vi "Init.vi"(8 "error in":errorcluster, 11 "object in":refnum<class "Camera Imaqdx CFG.lvclass">) -> (0 "error out":errorcluster, 3 "object out":refnum<class "Camera Imaqdx CFG.lvclass">)   [LabVIEW 2023, in "Camera Imaqdx CFG.lvclass"]
uses:
  Camera Imaqdx CFG.lvclass
  Camera Imaqdx CFG.lvclass/Camera Imaqdx CFG.ctl
  <vilib>/vision/driver/NI_Vision_Acquisition_Software.lvlib
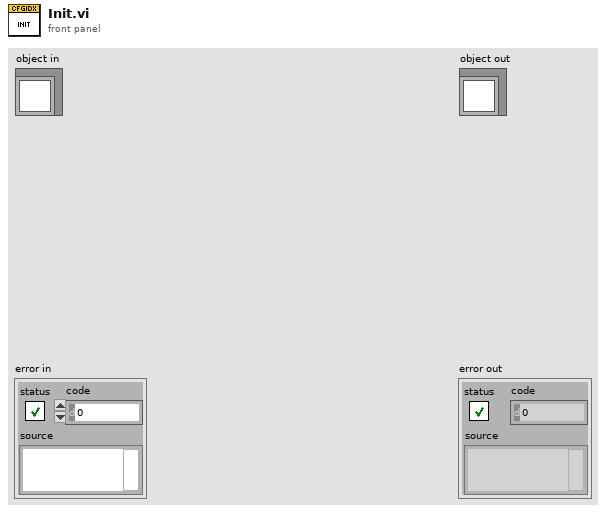
[diagram p1: front panel]
types:
  T1 = typedef "IMAQdx.ctl" = refnum<k21>
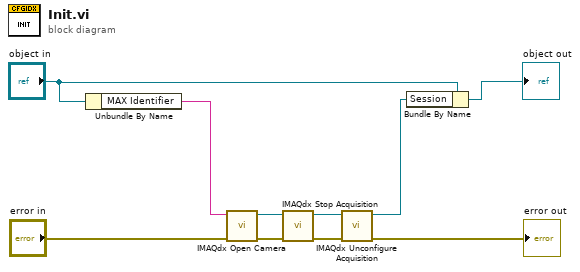
[diagram p0: block diagram]
diagram:
  n1 = Unbundle By Name("object in") -> ("MAX Identifier"=w3:string)
  n2 = call <vilib>:"IMAQdx Open Camera.vi"("error in"="error in", "Session In"=w3) -> ("error out"=w9:errorcluster, "Session Out"=w7:T1)  [unwired: 8 in]
  n3 = call <vilib>:"IMAQdx Stop Acquisition.vi"("error in"=w9, "Session In"=w7) -> ("error out"=w8:errorcluster, "Session Out"=w5:T1)  [unwired: 8 in]
  n4 = call <vilib>:"IMAQdx Unconfigure Acquisition.vi"("error in"=w8, "Session In"=w5) -> ("error out"=→"error out":errorcluster, "Session Out"=w4:T1)  [unwired: 8 in]
  n5 = Bundle By Name(cluster="object in", "Session"=w4) -> (→"object out":refnum<class "Camera Imaqdx CFG.lvclass">)
